vi "insert_edge_nodes.vi"(7 "edge type":refnum<class "Edge.lvclass">, 9 "node-b":refnum<class "Node.lvclass">, 10 "node-a":refnum<class "Node.lvclass">, 11 "graph":refnum<class "Graph.lvclass">) -> (1 "edge unchanged?":bool, 2 "edge already included?":bool, 3 "graph out":refnum<class "Graph.lvclass">, 5 "new edge":refnum<class "Edge.lvclass">)   [LabVIEW 2020, in "graph.lvlib" / "Graph.lvclass"]
uses:
  Graph.lvclass
  Node/Node.lvclass
  Edge/Edge.lvclass
  Graph.lvclass/Graph.ctl
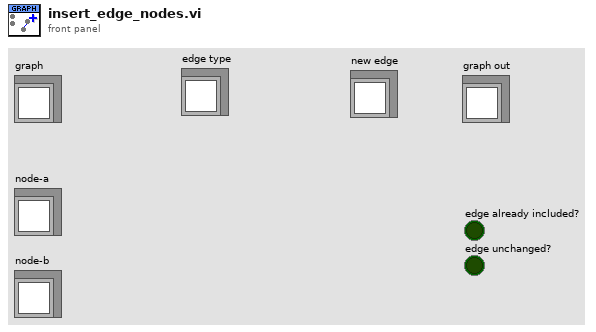
[diagram p1: front panel]
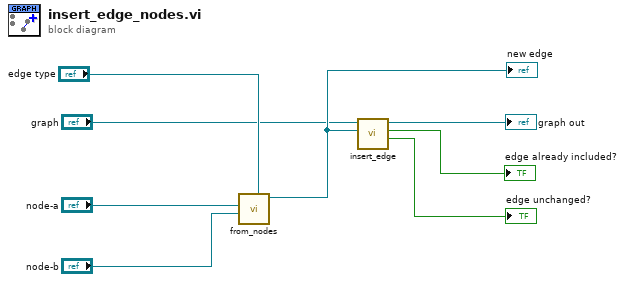
[diagram p0: block diagram]
diagram:
  n1 = call-dynamic "from_nodes.vi"("edge type"="edge type", "node-b"="node-b", "node-a"="node-a") -> ("new edge"=w5:refnum<class "Edge.lvclass">)  [unwired: 8 in]
  "new edge" <- w5
  n2 = call-dynamic "insert_edge.vi"("edge"=w5, "graph"="graph") -> ("edge unchanged?"=→"edge unchanged?":bool, "edge already included?"=→"edge already included?":bool, "graph out"=→"graph out":refnum<class "Graph.lvclass">)  [unwired: 7 in]
